vi "util_camProperties.vi"() -> ()   [LabVIEW 2013]
uses:
  <vilib>/userdefined/High Color/IMAQdx.ctl
  <vilib>/vision/driver/IMAQdx.llb/IMAQdx Attribute Type.ctl
  <vilib>/vision/driver/NI_Vision_Acquisition_Software.lvlib
panel:
  in  "?":bool
  out "Video Modes":T1(array[cluster])
  out "Attribute Information Array":T3(array[cluster])
  out "error out":errorcluster
  out "Image":T4(plugin-control)
  in  "Camera":T5="cam0"
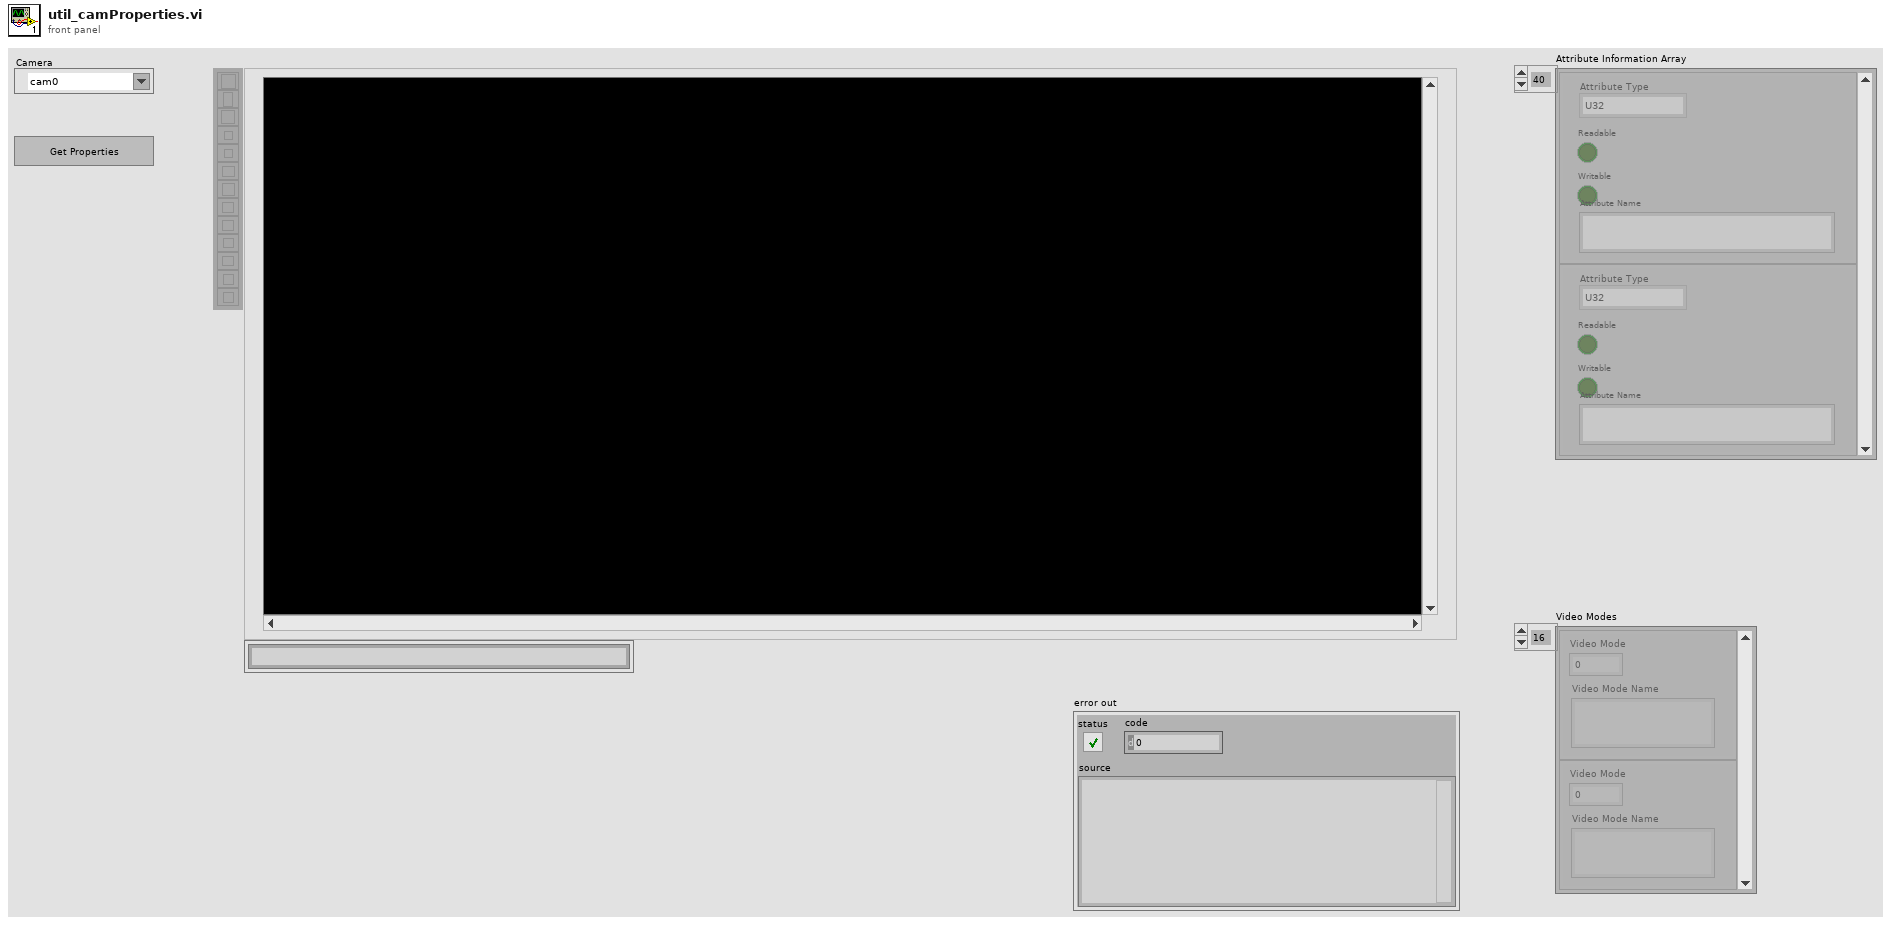
[diagram p1: front panel]
types:
  T1 = cluster{"Video Mode":u32, "Video Mode Name":string}[]
  T2 = typedef "NI_Vision_Acquisition_Software.lvlib/IMAQdx Attribute Type.ctl" = enum32{"U32", "I64", "DBL", "String", "Enum", "Bool", "Command"}
  T3 = cluster{"Attribute Type":T2, "Readable":bool, "Writable":bool, "Attribute Name":string}[]
  T4 = typedef "IMAQ Image.ctl" = refnum<image>
  T5 = typedef "IMAQdx.ctl" = refnum<k21>
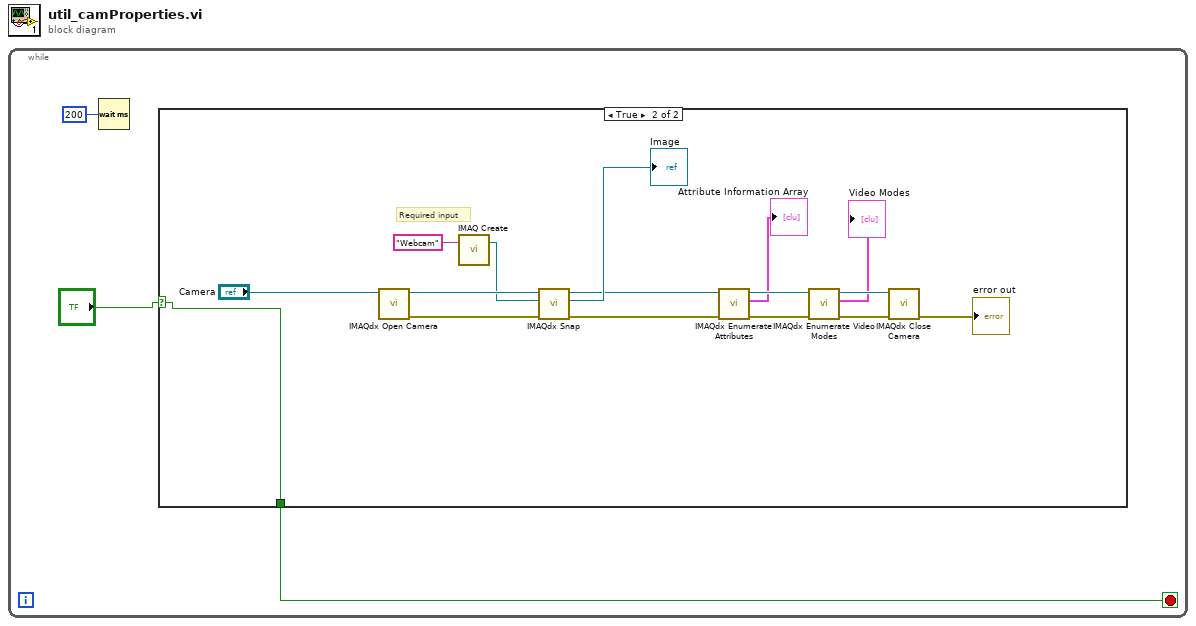
[diagram p0: block diagram]
diagram:
  n1 = while {
    stop <- w2 stop-if-true
    n2 = Wait (ms)(milliseconds to wait=u32 200) -> ()  [unwired: 1 out]
    n3 = case shown="True" "?" {
      selector: "?" -> [w4 w5]
      tunnel: [w4 w5] -> w2
      frame False {
      }
      frame True {
        # "Required input"
        n4 = call <vilib>:"IMAQdx Open Camera.vi"("Session In"="Camera") -> ("error out"=w19:errorcluster, "Session Out"=w20:T5)  [unwired: 9 in]
        n5 = call "IMAQ Create"("Image Name"="Webcam") -> ("New Image"=w18:T4)  [unwired: 4 in, 1 out]
        n6 = call <vilib>:"IMAQdx Snap.vi"("error in"=w19, "Image In"=w18, "Session In"=w20) -> ("error out"=w12:errorcluster, "Image Out"=→"Image":T4, "Session Out"=w8:T5)  [unwired: 6 in]
        n7 = call <vilib>:"IMAQdx Enumerate Attributes.vi"("error in"=w12, "Session In"=w8) -> ("error out"=w13:errorcluster, "Attribute Information Array"=→"Attribute Information Array":T3, "Session Out"=w9:T5)  [unwired: 7 in]
        n8 = call <vilib>:"IMAQdx Enumerate Video Modes.vi"("error in"=w13, "Session In"=w9) -> ("error out"=w14:errorcluster, "Video Modes"=→"Video Modes":T1, "Session Out"=w10:T5)  [unwired: 6 in, 1 out]
        n9 = call <vilib>:"IMAQdx Close Camera.vi"("error in"=w14, "Session In"=w10) -> ("error out"=→"error out":errorcluster)  [unwired: 9 in]
      }
    }
  }
